vi "Regular Autonomous (subVI of AutoIndep).vi"() -> ()   [LabVIEW 2013]
uses:
  2014 Target Detection/TargetType.ctl
panel:
  in  "Hot":i32
  in  "Not hot":i32=50
  in  "Down break":dbl=10.0 format="%#_13g"
  in  "Move":i32=500
  out "Goal State":T1
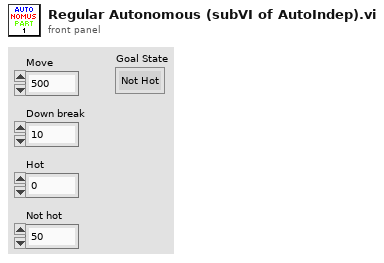
[diagram p1: front panel]
types:
  T1 = typedef "TargetType.ctl" = enum16{"Not Hot", "Hot"}
  T2 = cluster{"Scores":cluster{"Total":dbl, "Left":dbl, "Right":dbl, "Ratio":dbl, "Vertical":dbl, "index":i32, "State":T1}, "Verticals":cluster{"Horizontal?":bool, "Aspect Score":dbl, "Rect Score":dbl, cluster{"Left":dbl, "Top":dbl, "Right":dbl, "Bottom":dbl}, "Equiv H":dbl, "Equiv V":dbl}, "Horizontals":cluster{"Horizontal?":bool, "Aspect Score":dbl, "Rect Score":dbl, cluster{"Left":dbl, "Top":dbl, "Right":dbl, "Bottom":dbl}, "Equiv H":dbl, "Equiv V":dbl}, "Distance ft":dbl, "Center":cluster{"X":dbl, "Y":dbl}}[]
  T3 = cluster{"Scores":cluster{"Total":dbl, "Left":dbl, "Right":dbl, "Ratio":dbl, "Vertical":dbl, "index":i32, "State":T1}, "Verticals":cluster{"Horizontal?":bool, "Aspect Score":dbl, "Rect Score":dbl, cluster{"Left":dbl, "Top":dbl, "Right":dbl, "Bottom":dbl}, "Equiv H":dbl, "Equiv V":dbl}, "Horizontals":cluster{"Horizontal?":bool, "Aspect Score":dbl, "Rect Score":dbl, cluster{"Left":dbl, "Top":dbl, "Right":dbl, "Bottom":dbl}, "Equiv H":dbl, "Equiv V":dbl}, "Distance ft":dbl, "Center":cluster{"X":dbl, "Y":dbl}}
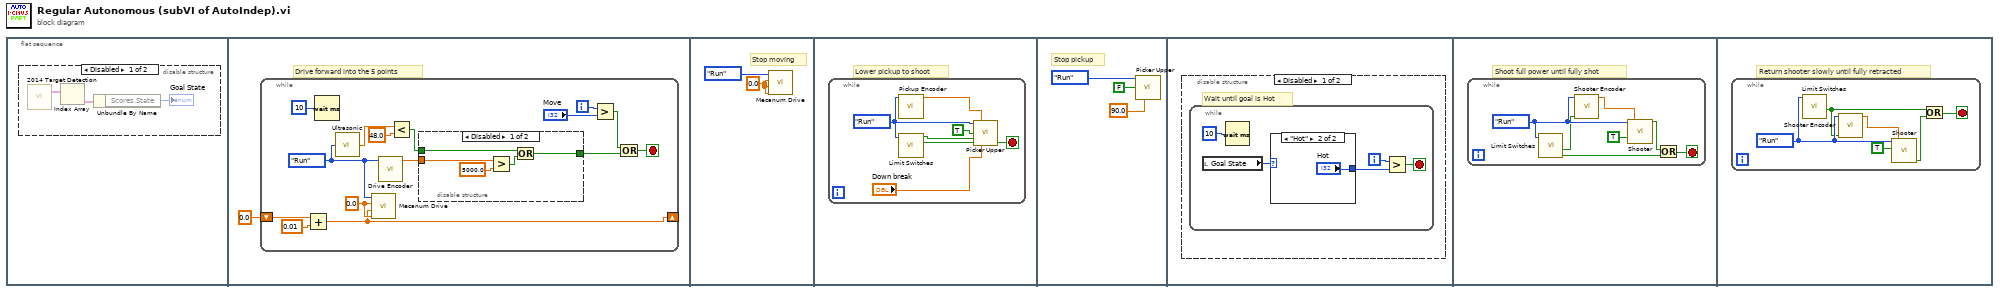
[diagram p0: block diagram]
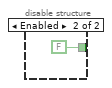
[diagram p3: hidden frame]
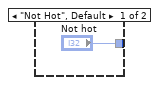
[diagram p4: hidden frame]
diagram:
  n1 = flat-sequence {
    frame #0 {
      n2 = disable-structure shown="Disabled" {
        frame Disabled {
          n3 = call "2014 Target Detection.vi"() -> ("Target Info"=w3:T2)  [unwired: 1 in, 1 out]
          n4 = Index Array(array=w3) -> (element=w2:T3)  [unwired: 1 in]
          n5 = Unbundle By Name(w2) -> ("Scores.State"=→"Goal State":T1)
        }
        frame Enabled {
        }
      }
    }
    frame #1 {
      # "Drive forward into the 5 points"
      n6 = while {
        shift-right: [w7] -> _
        shift-left: 0.0 ("Strafing") -> [w9]
        i -> [w19]
        stop <- w12 stop-if-true
        w16 = 0.0 ("Strafing")
        w6 = enum16{"Open", "Run", "End"}."Run" ("State Control")
        n7 = Add(x=w9, y=0.01) -> (x+y=w7:dbl)
        n8 = Wait (ms)(milliseconds to wait=u32 10) -> ()  [unwired: 1 out]
        n9 = call "Ultrasonic.vi"("State Control"=w6) -> ("Distance (in.)"=w15:dbl)
        n10 = call "Mecanum Drive.vi"("Turn"=w16, "Forward/Backward"=w7, "Strafe"=w16, "State Control"=w6) -> ()  [unwired: 4 in]
        n11 = call "Drive Encoder.vi"("State Control"=w6) -> ("Encoder Degrees"=w5:dbl)  [unwired: 3 in, 3 out]
        n12 = Less?(x=w15, y=48.0) -> (x < y?=w10:bool)
        n13 = disable-structure shown="Disabled" {
          disable-tunnel: [w20 FALSE] -> w11
          disable-tunnel: w10 -> [w21 _]
          disable-tunnel: w5 -> [w24 _]
          frame Disabled {
            n14 = Greater?(x=w24, y=5000.0) -> (0:w22:bool)
            n15 = Or(x=w21, y=w22) -> (x .or. y?=w20:bool)
          }
          frame Enabled {
          }
        }
        n16 = Greater?(x=w19, y="Move") -> (0:w13:bool)
        n17 = Or(x=w13, y=w11) -> (x .or. y?=w12:bool)
      }
    }
    frame #2 {
      w26 = 0.0 ("F/R")
      # "Stop moving"
      n18 = call "Mecanum Drive.vi"("Turn"=w26, "Forward/Backward"=w26, "Strafe"=w26, "State Control"=enum16{"Open", "Run", "End"}."Run") -> ()  [unwired: 4 in]
    }
    frame #3 {
      # "Lower pickup to shoot"
      n19 = while {
        stop <- w34 stop-if-true
        w32 = enum16{"Open", "Run", "End"}."Run" ("State Control")
        n20 = call "Pickup Encoder.vi"("State Control"=w32) -> ("Encoder Degrees"=w31:dbl)  [unwired: 3 in, 3 out]
        n21 = call "Limit Switches.vi"("State Control"=w32) -> ("Picker Upper Bottom"=w33:bool, "Picker Upper Top"=w29:bool)  [unwired: 7 in, 2 out]
        n22 = call "Picker Upper.vi"("State Control"=w32, "Encoder"=w31, "Down"=TRUE, "Top limit"=w29, "Bottom Limit"=w33, "Down break"="Down break") -> ("Fully down?"=w34:bool)  [unwired: 8 in, 1 out]
      }
    }
    frame #4 {
      # "Stop pickup"
      n23 = call "Picker Upper.vi"("State Control"=enum16{"Open", "Run", "End"}."Run", "Down"=FALSE, "Down break"=90.0) -> ()  [unwired: 11 in, 2 out]
    }
    frame #5 {
      n24 = disable-structure shown="Disabled" {
        frame Disabled {
          # "Wait until goal is Hot"
          n25 = while {
            i -> [w42]
            stop <- w41 stop-if-true
            n26 = local read "Goal State"() -> (w39:T1)
            n27 = Wait (ms)(milliseconds to wait=u32 10) -> ()  [unwired: 1 out]
            n28 = case shown="\"Hot\"" w39 {
              tunnel: ["Not hot" "Hot"] -> w38
              frame "Not Hot", Default {
              }
              frame "Hot" {
              }
            }
            n29 = Greater?(x=w42, y=w38) -> (0:w41:bool)
          }
        }
        frame Enabled {
        }
      }
    }
    frame #6 {
      # "Shoot full power until fully shot"
      n30 = while {
        stop <- w48 stop-if-true
        w51 = enum16{"Open", "Run", "End"}."Run" ("State Control")
        n31 = call "Limit Switches.vi"("State Control"=w51) -> ("Shooter Top"=w49:bool, "Shooter Bottom"=w46:bool)  [unwired: 7 in, 2 out]
        n32 = call "Shooter Encoder.vi"("Reset Encoder?"=w46, "State Control"=w51) -> ("Encoder Degrees"=w47:dbl)  [unwired: 2 in, 3 out]
        n33 = call "Shooter.vi"("State Control"=w51, "4 ft"=TRUE, "Encoder"=w47) -> ("Fully shot?"=w50:bool)  [unwired: 15 in, 1 out]
        n34 = Or(x=w50, y=w49) -> (x .or. y?=w48:bool)
      }
    }
    frame #7 {
      # "Return shooter slowly until fully retracted"
      n35 = while {
        stop <- w54 stop-if-true
        w57 = enum16{"Open", "Run", "End"}."Run" ("State Control")
        n36 = call "Limit Switches.vi"("State Control"=w57) -> ("Shooter Bottom"=w53:bool)  [unwired: 7 in, 3 out]
        n37 = call "Shooter Encoder.vi"("Reset Encoder?"=w53, "State Control"=w57) -> ("Encoder Degrees"=w56:dbl)  [unwired: 2 in, 3 out]
        n38 = call "Shooter.vi"("State Control"=w57, "Return"=TRUE, "Encoder"=w56) -> ("Fully retracted?"=w55:bool)  [unwired: 15 in, 1 out]
        n39 = Or(x=w53, y=w55) -> (x .or. y?=w54:bool)
      }
    }
  }
